vi "KundtsTube.vi"() -> ()   [LabVIEW 2014]
uses:
  <vilib>/imath/engines/lvmath2/RunTimeEngine/Managers/WorkSpace/UID Generator.vi
  <vilib>/imath/engines/lvmath2/RunTimeEngine/RunTimeType/NIMS_RunTimeType_From StrictType (excl LVString).vi
  <instcachedir>/0/NIMS_RunTimeType_From StrictType (excl LVString)_15A5391EEA9C4AACB9955AC755B83D29.lvgen/NIMS_RunTimeType_From StrictType (excl LVString)_15A5391EEA9C4AACB9955AC755B83D29_000.vi
  <vilib>/imath/engines/lvmath2/RunTimeEngine/LocalVariableDefStatement/MC_LocalVariableDefStatement_Display.vi
  <vilib>/imath/engines/lvmath2/RunTimeEngine/Managers/SymbolTable/Clear UID.vi
  <vilib>/imath/engines/lvmath2/RunTimeEngine/NodeEndStatement/NIMS_NodeEndStatement_Output.vi
  <instcachedir>/0/NIMS_NodeEndStatement_Output_53EC0D466D134D7ABD903AC30B43404B.lvgen/NIMS_NodeEndStatement_Output_53EC0D466D134D7ABD903AC30B43404B_005.vi
  <vilib>/imath/engines/lvmath2/RunTimeEngine/ErrorHandling/NIMS_Finalize Error.vi
  <vilib>/imath/engines/lvmath2/RunTimeEngine/Managers/SymbolTable/NIMS_WorkSpace.lvlib
panel:
  in  "stop":bool
  out "Gain vs Frequnency":cluster{"Y":dbl[], "Y":dbl[]}[](graph)
  out "Output":cluster{"Frequency":dbl, "RMS":dbl}={"Frequency"=10000.0, "RMS"=0.010773391494968265}
  out "data":dynamicdata(graph)=[{"t0"=timestamp(3497991676.4311037 s since 1904-01-01), "dt"=9.999999999999972e-06, "Y"=array[100000 elements], "attributes"=variant("NI_ChannelName"=variant(string "Voltage"), "NI_UnitDescription"=variant(string "Volts"))}]
  in  "Waveform Digitization":T1={"Sampling Rate (Hz)"=100000.0, "# of Samples"=100000.0}
  in  "Amplitude":dbl=2.0
  in  "Array Parameters":T2={"Minimum"=10.0, "Maximum"=10000.0, "# of Points"=1999.0, "Spacing"=0} {"Spacing" items=["Linear", "Logarithmic"]}
  in  "Tab Control":enum32{"Sweep", "Single"}(tab)
  in  "Dwell Time (sec)":u32=1
  in  "Single Frequency":dbl=100.0
  # "This will sweep from in to max, \npausing by the dwell time after\neach increments."
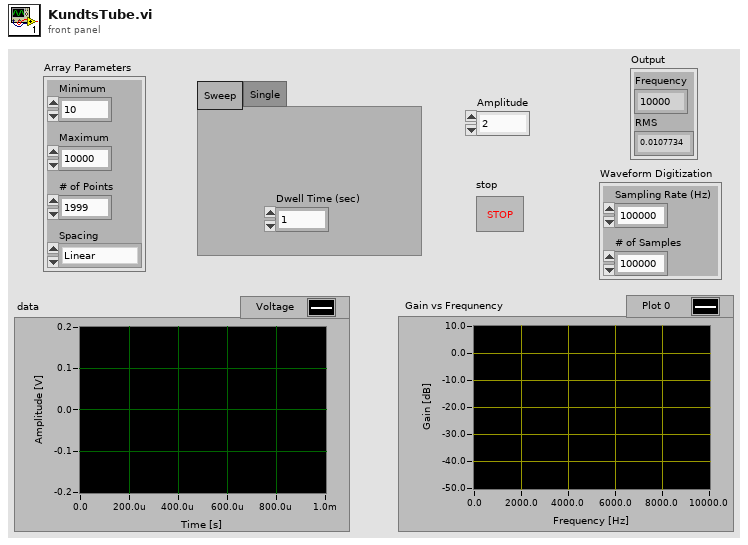
[diagram p1: front panel]
types:
  T1 = cluster{"Sampling Rate (Hz)":dbl, "# of Samples":dbl}
  T2 = cluster{"Minimum":dbl, "Maximum":dbl, "# of Points":dbl, "Spacing":u16}
  T3 = enum16{"open", "replace", "create", "open or create", "replace or create", "replace or create with confirmation"}
  T4 = cluster{"Single Frequency":dbl, "AC estimate (Vrms)":dbl}
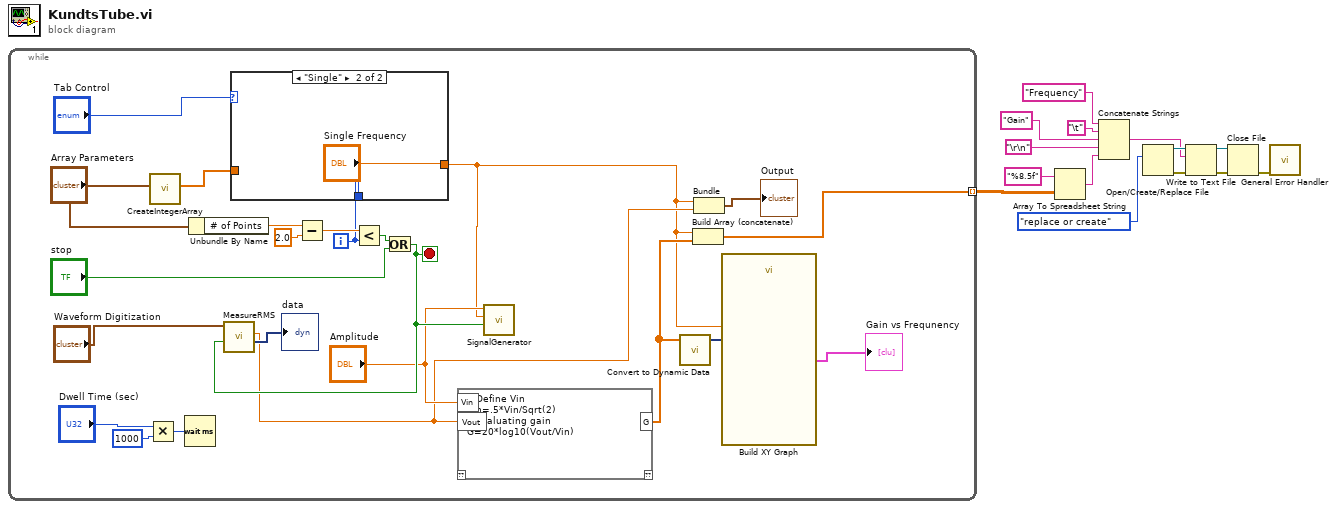
[diagram p0: block diagram]
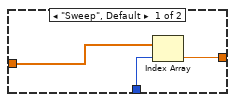
[diagram p2: hidden frame]
diagram:
  n1 = while {
    tunnel: [w19] -> w1 mode=indexing
    i -> [w15]
    stop <- w26 stop-if-true
    n2 = Multiply(x="Dwell Time (sec)", y=u32 1000) -> (x*y=w32:u32)
    n3 = call "CreateIntegerArray.vi"("Array Parameters"="Array Parameters") -> ("Out Array"=w30:dbl[])  [unwired: 10 in]
    n4 = Wait (ms)(milliseconds to wait=w32) -> ()  [unwired: 1 out]
    n5 = Unbundle By Name("Array Parameters") -> ("# of Points"=w23:dbl)
    n6 = case shown="\"Single\"" "Tab Control" {
      tunnel: [w101 "Single Frequency"] -> w16
      tunnel: w30 -> [w102 _]
      tunnel: w15 -> [w100 _]
      frame "Sweep", Default {
        n7 = Index Array(array=w102, index=w100) -> (element=w101:dbl)
      }
      frame "Single" {
      }
    }
    n8 = Subtract(x=w23, y=2.0) -> (x-y=w22:dbl)
    n9 = Less?(x=w22, y=w15) -> (x < y?=w24:bool)
    n10 = Or(x=w24, y="stop") -> (x .or. y?=w26:bool)
    n11 = call "MeasureRMS.vi"("stop"=w26, "input cluster"="Waveform Digitization") -> ("data"=→"data":dynamicdata, "AC estimate (Vrms)"=w18:dbl)  [unwired: 5 in, 1 out]
    n12 = mathscript code="%Define Vin\nVin=.5*Vin/Sqrt(2)\n%Evaluating gain \nG=20*log10(Vout/Vin)"("Vout"=w18, "Vin"="Amplitude") -> ("G"=w17:dbl[])  [unwired: 1 in, 1 out]
    n13 = call "SignalGenerator.vi"("stop"=w26, "Frequency"=w16, "Amplitude"="Amplitude") -> ()  [unwired: 4 in, 1 out]
    n14 = call "Convert to Dynamic Data"("Array"=w17) -> ("Dynamic Data Type"=w29:dynamicdata)  [unwired: 3 in]
    n15 = Build Array (concatenate)(w16, w17) -> (w19:dbl[])
    n16 = Bundle("Single Frequency"=w16, "AC estimate (Vrms)"=w18) -> (→"Output":T4)  [unwired: 1 in]
    n17 = call "Build XY Graph"("Y Input"=w29, "X Input"=w16) -> ("XY Graph"=→"Gain vs Frequnency":cluster{"X":dbl[], "Y":dbl[]}[])  [unwired: 8 in, 1 out]
  }
  n18 = Array To Spreadsheet String(array=w1, 3:"%8.5f" ("format string")) -> (spreadsheet string=w4:string)  [unwired: 1 in]
  n19 = Concatenate Strings("Frequency" ("string"), "\t", "Gain" ("string"), "\r\n", w4) -> (w2:string)
  n20 = Open/Create/Replace File(operation (0:open)=T3."replace or create") -> (refnum out=w14:refnum<file>, error out=w11:errorcluster)  [unwired: 5 in, 1 out]
  n21 = Write to Text File(file (use dialog)=w14, text=w2, error in=w11) -> (refnum out=w13:refnum<file>, error out=w12:errorcluster)  [unwired: 1 in, 1 out]
  n22 = Close File(refnum=w13, error in=w12) -> (error out=w10:errorcluster)  [unwired: 1 out]
  n23 = call <vilib>:"General Error Handler.vi"("error in (no error)"=w10) -> ()  [unwired: 10 in, 5 out]
